vi "generate xyz data.vi"(6 "yrange":dbl, 7 "xrange":dbl, 8 "error in (no error)":errorcluster, 9 "n":i32, 10 "zdata":dbl, 11 "xydata":dbl) -> (0 "error out":errorcluster, 1 "function return":i32, 2 "zdata out":dbl, 3 "xydata out":dbl)   [LabVIEW 2014, in "libgwyscan.lvlib"]
doc: "GWYSCANDLL_API int generate_xyz_data(double *xydata, double *zdata, int n, double xrange, double yrange);"
uses:
  <userlib>/libgwyscan/libgwyscan.lvlib
  <userlib>/libgwyscan/libgwyscan.dll
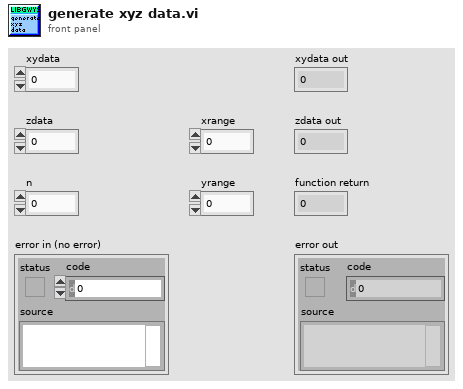
[diagram p1: front panel]
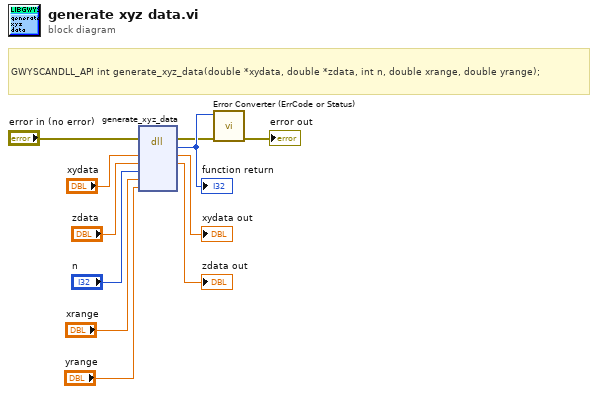
[diagram p0: block diagram]
diagram:
  # "GWYSCANDLL_API int generate_xyz_data(double *xydata, double *zdata, int n, double xrange, double yrange);"
  n1 = dll-call lib="C:/Program Files/National Instruments/LabVIEW 2014/user.lib/libgwyscan/libgwyscan.*" fn="generate_xyz_data"(error in="error in (no error)", "xydata"="xydata", "zdata"="zdata", "n"="n", "xrange"="xrange", "yrange"="yrange") -> (error out=w2:errorcluster, w11:i32, "xydata"=→"xydata out":dbl, "zdata"=→"zdata out":dbl)  [unwired: 5 in, 1 out]
  "function return" <- w11
  n2 = call <userlib>:"Error Converter (ErrCode or Status).vi"("error in (no error)"=w2, "error code"=w11) -> ("error out"=→"error out":errorcluster)  [unwired: 9 in]
